vi "ROI group-Vis window refresh signal.vi"(8 "error in (no error)":errorcluster) -> (0 "error out":errorcluster)   [LabVIEW 2017]
uses:
  ROI grouping window/Globals/gl_ROI grp window globals.vi
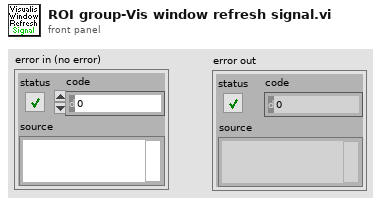
[diagram p1: front panel]
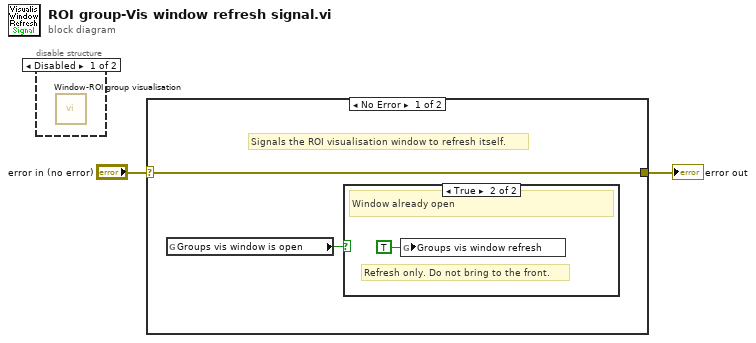
[diagram p0: block diagram]
diagram:
  n1 = disable-structure shown="Disabled" {
    frame Disabled {
      n2 = call "Window-ROI group visualisation.vi"() -> ()  [unwired: 11 in, 1 out]
    }
    frame Enabled {
    }
  }
  n3 = case shown="No Error" "error in (no error)" {
    selector: "error in (no error)" -> [w4 w6]
    tunnel: [w4 w6] -> w1
    frame No Error {
      # "Signals the ROI visualisation window to refresh itself."
      n4 = global read "gl_ROI grp window globals.vi" "Groups vis window is open"() -> (w3:bool)
      n5 = case shown="True" w3 {
        frame False {
          # "Window is not open"
        }
        frame True {
          # "Refresh only. Do not bring to the front."
          # "Window already open"
          n6 = global write "gl_ROI grp window globals.vi" "Groups vis window refresh"(TRUE ("Groups vis window refresh")) -> ()
        }
      }
    }
    frame Error {
    }
  }
  "error out" <- w1
